vi "Session Daemon Async.vi"(9 "Engine Notifier":refnum<notifier>, 10 "TS License Type":T1, 11 "Dev Debug?":bool) -> ()   [LabVIEW 2020, in "TSnax.lvlib" / "Engine.lvclass"]
uses:
  Engine.lvclass
  TS License Type.ctl
  Daemon State.ctl
  UIMessage Callbacks.ctl
  UIMessage Callback.ctl
  UIMsg Callback VI.ctl
  UIMsg.ctl
  Ref Data.ctl
  PropertyObject/PropertyObject.lvclass
  SequenceFile/SequenceFile.lvclass
  Engine.lvclass/Engine.ctl
  SequenceFile Response.ctl
  VariableContainer Response.ctl
  Execution Response.ctl
  Execution/Execution.lvclass
  Report Response.ctl
  Report/Report.lvclass
  UIMessage/UIMessage.lvclass
  TSnax.lvlib
panel:
  out "Log":string
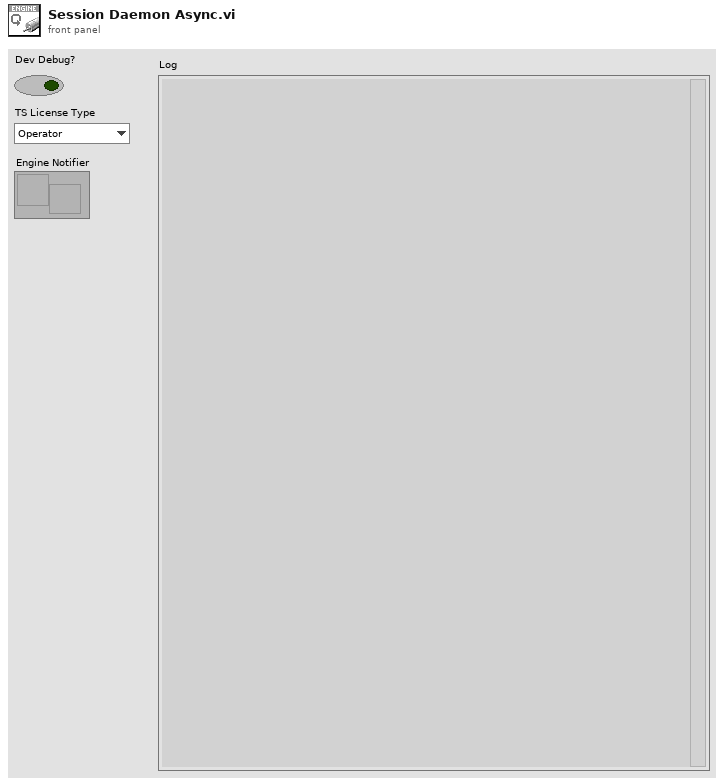
[diagram p1: front panel]
types:
  T1 = typedef "TSnax.lvlib/TS License Type.ctl" = enum16{"Operator", "CustomEditor", "SequenceEditor"}
  T2 = enum32{"invalid app kind", "Development System", "Run Time System", "Student Edition", "Embedded LabVIEW", "Evaluation", "Custom"}
  T3 = typedef "TSnax.lvlib/Engine.lvclass/Daemon State.ctl" = enum16{"Init", "Run", "Close"}
  T4 = typedef "TSnax.lvlib/Engine.lvclass/Ref Data.ctl" = cluster{"Station Globals":refnum<class "PropertyObject.lvclass">, "Station Model":refnum<class "SequenceFile.lvclass">, "Trace Delay":u32, "Execution Map":map{i32, refnum<class "Execution.lvclass">}}
  T5 = typedef "TSnax.lvlib/Engine.lvclass/UIMessage Callbacks.ctl" = cluster{"Callbacks":T6[], "ID Map":map{T8, i32[]}}
  T6 = typedef "TSnax.lvlib/Engine.lvclass/UIMessage Callback.ctl" = cluster{"VI":T7, "Owner":refnum<class>, "User Data":variant, "IDs":T8[]}
  T7 = typedef "TSnax.lvlib/Engine.lvclass/UIMsg Callback VI.ctl" = refnum<vi>
  T8 = typedef "TSnax.lvlib/UIMsg.ctl" = enum16{"Unknown", "BreakOnUserRequest", "BreakOnBreakpoint", "BreakOnRunTimeError", "Trace", "TerminatingExecution", "AbortingExecution", "KillingExecutionThreads", "EndExecution", "ShutDownComplete", "StartExecution", "ProgressPercent", "ProgressText", "StartInteractiveExecution", "EndInteractiveExecution", "TerminatingInteractiveExecution", "TerminationCancelled", "ResumeFromBreak", "StartFileExecution", "EndFileExecution", "ShutDownCancelled", "LocalizationSettingChanged", "OpenWindows", "TileWindows", "CascadeWindows", "ReportChanged", "CloseWindows", "RefreshWindows", "ClientFileChanged", "DisplayReport", "ModelState_Initializing", "ModelState_Waiting", "ModelState_Identified", "ModelState_BeginTesting", "ModelState_TestingComplete", "ModelState_PostProcessingComplete", "ModelState_EnabledStateSet", "ReportLocationChanged", "GotoLocation", "PushUndoItem", "OutputMessages", "TypePaletteFileListChanged", "NonTerminatingThreadsArePreventingTermination", "ModelState_PostProcessing", "ReportCollectionChanged", "RuntimeError"}
  T9 = enum32{"Invalid", "Standard", "Closed", "Hidden", "Minimized", "Maximized"}
  T10 = typedef "TSnax.lvlib/Engine.lvclass/SequenceFile Response.ctl" = cluster{"SequenceFile":refnum<class "SequenceFile.lvclass">, "Error":errorcluster}
  T11 = typedef "TSnax.lvlib/Engine.lvclass/VariableContainer Response.ctl" = cluster{"PropertyObject":refnum<class "PropertyObject.lvclass">, "Error":errorcluster}
  T12 = typedef "TSnax.lvlib/Engine.lvclass/Execution Response.ctl" = cluster{"Execution":refnum<class "Execution.lvclass">, "Error":errorcluster}
  T13 = typedef "TSnax.lvlib/Engine.lvclass/Report Response.ctl" = cluster{"Report":refnum<class "Report.lvclass">, "Error":errorcluster}
  T14 = typedef "TSnax.lvlib/File Load Options.ctl" = cluster{"Use Search Dirs? (T)":bool, "Conflict as Error? (T)":bool, "Check Station Model? (F)":bool, "Preload Modules? (T)":bool, "Skip Load Callback? (F)":bool, "Reload if Loaded? (F)":bool}
  T15 = typedef "TSnax.lvlib/Engine.lvclass/VariableContainer Type.ctl" = enum16{"StationGlobals", "TemporaryGlobals", "NewPropertyObject", "SubProperty"}
  T16 = typedef "TSnax.lvlib/Execution Options.ctl" = cluster{"Use Default Model (T)":bool, "Release Related References (T)":bool}
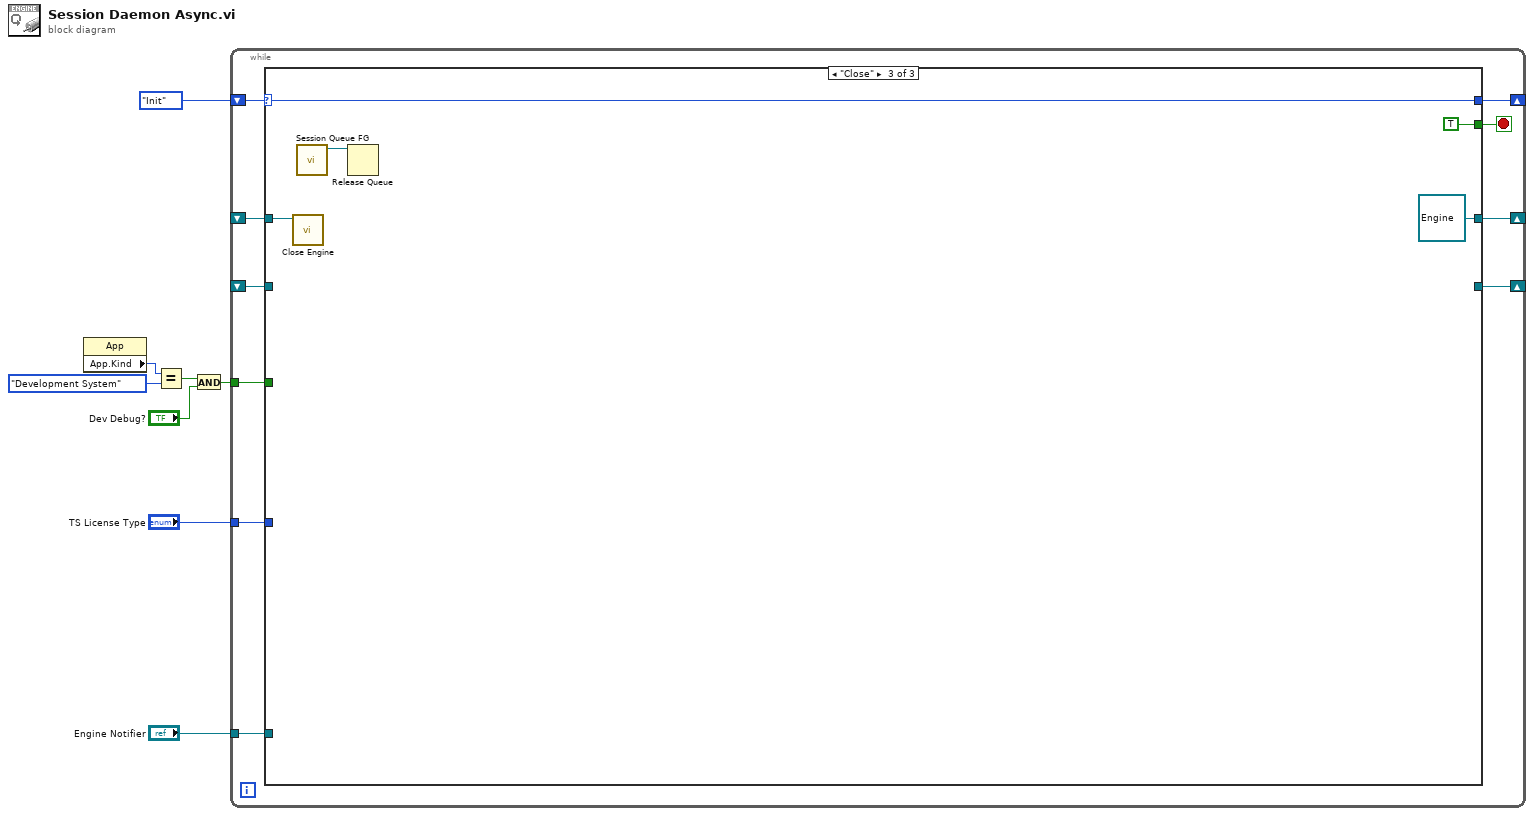
[diagram p0: block diagram]
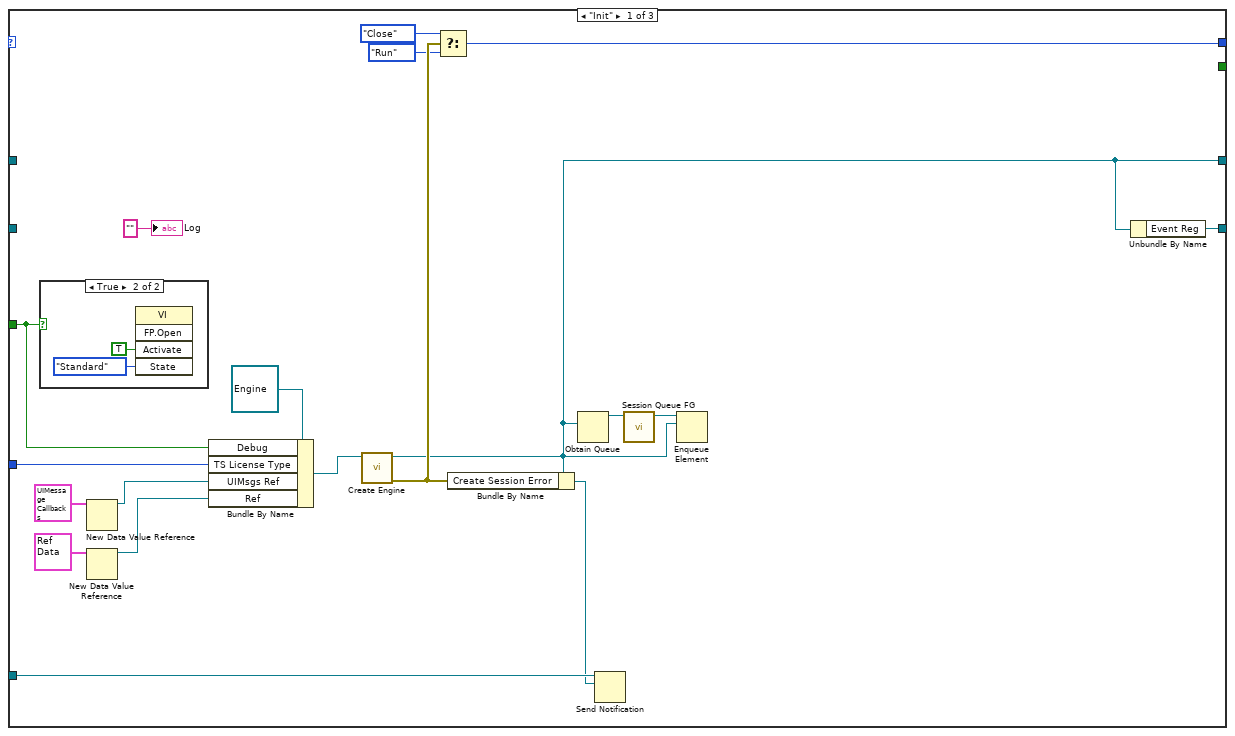
[diagram p2: hidden frame]
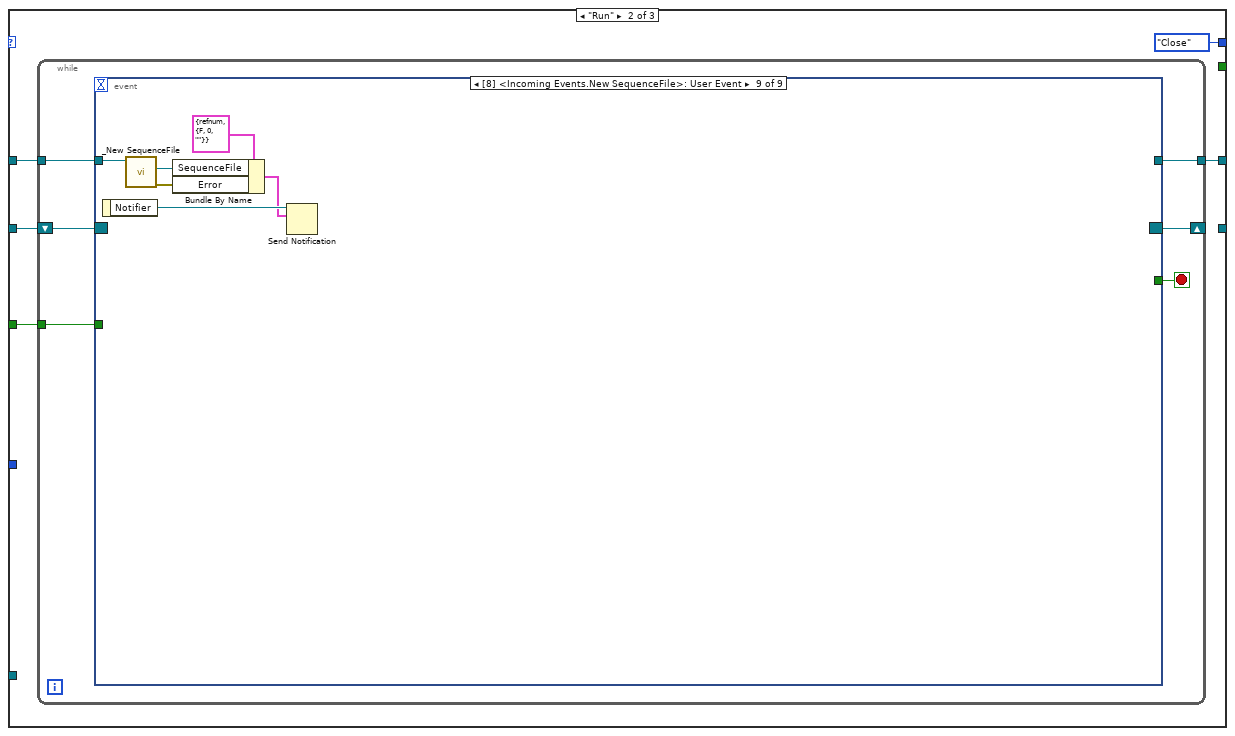
[diagram p4: hidden frame]
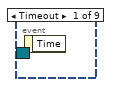
[diagram p5: hidden frame]
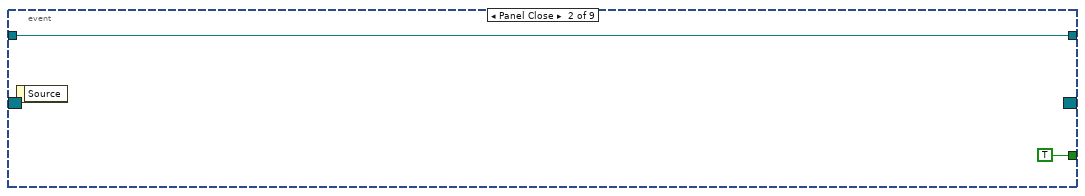
[diagram p6: hidden frame]
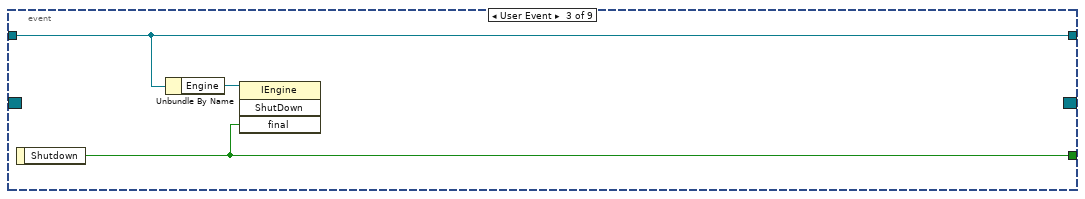
[diagram p7: hidden frame]
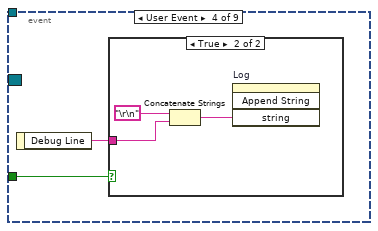
[diagram p8: hidden frame]
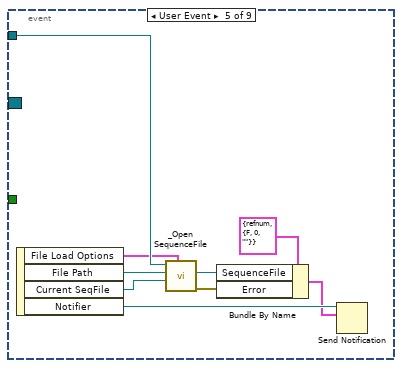
[diagram p10: hidden frame]
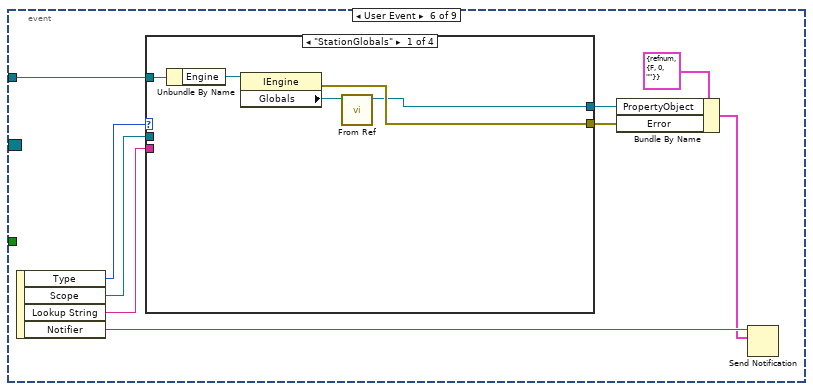
[diagram p11: hidden frame]
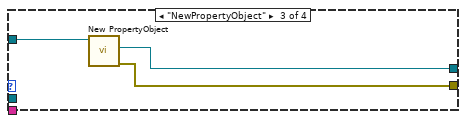
[diagram p13: hidden frame]
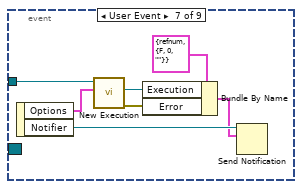
[diagram p15: hidden frame]
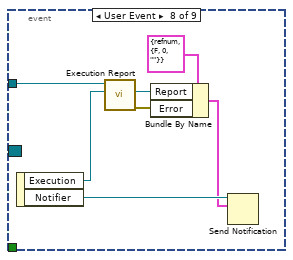
[diagram p16: hidden frame]
diagram:
  n1 = property class="App"() -> ("App.Kind"=w5:T2)  [unwired: 2 in, 2 out]
  n2 = Equal?(x=w5, y=T2."Development System") -> (x = y?=w3:bool)
  n3 = And(x=w3, y="Dev Debug?") -> (x .and. y?=w2:bool)
  n4 = while {
    shift-right: [w17] -> _
    shift-left: Daemon_State."Init" ("Daemon State") -> [w18]
    tunnel: "TS License Type" -> [w15]
    tunnel: "Engine Notifier" -> [w14]
    tunnel: w2 -> [w13]
    shift-right: [w12] -> _
    shift-left: _ -> [w11]
    shift-right: [w10] -> _
    shift-left: _ -> [w9]
    stop <- w16 stop-if-true
    n5 = case shown="\"Close\"" w18 {
      selector: w18 -> [_ _ w111]
      tunnel: [w30 Daemon_State."Close" ("Daemon State") w111] -> w17
      tunnel: [_ _ TRUE] -> w16
      tunnel: w15 -> [w35 _ _]
      tunnel: w14 -> [w33 _ _]
      tunnel: w13 -> [w28 w42 _]
      tunnel: [w24 w41 refnum<class "Engine.lvclass"> refnum ("Engine out")] -> w12
      tunnel: w11 -> [_ w43 w108]
      tunnel: [w27 _ _] -> w10
      tunnel: w9 -> [_ w40 _]
      frame "Init" {
        n6 = case shown="True" w28 {
          frame False {
          }
          frame True {
            n7 = invoke class="VI" method="FP.Open"("Activate"=TRUE ("Activate?"), "State"=T9."Standard") -> ()  [unwired: 3 in, 5 out]
          }
        }
        n8 = New Data Value Reference(data value=T5 {"Callbacks"=[], "ID Map"={}} ("UIMessage Callbacks")) -> (data value reference=w21:refnum<data-value>)  [unwired: 1 in, 1 out]
        n9 = New Data Value Reference(data value=T4 {"Station Globals"=refnum, "Station Model"=refnum, "Trace Delay"=0, "Execution Map"={}} ("Ref Data")) -> (data value reference=w19:refnum<data-value>)  [unwired: 1 in, 1 out]
        n10 = Bundle By Name(cluster=refnum<class "Engine.lvclass"> refnum ("TSnax.lvlib:Engine.lvclass"), "Debug"=w28, "TS License Type"=w35, "UIMsgs Ref"=w21, "Ref"=w19) -> (w34:refnum<class "Engine.lvclass">)
        n11 = call "Create Engine.vi"("Engine in"=w34) -> ("error out"=w37:errorcluster, "Engine out"=w24:refnum<class "Engine.lvclass">)  [unwired: 9 in]
        n12 = Select(t=Daemon_State."Close" ("Daemon State"), s=w37, f=Daemon_State."Run" ("Daemon State")) -> (s? t:f=w30:T3)
        n13 = Bundle By Name(cluster=w24, "Create Session Error"=w37) -> (w32:refnum<class "Engine.lvclass">)
        n14 = Obtain Queue(element data type=w24) -> (queue out=w26:refnum<queue>)  [unwired: 4 in, 2 out]
        n15 = Send Notification(notification=w32, notifier=w33) -> ()  [unwired: 1 in, 2 out]
        n16 = call "Session Queue FG.vi"("Session Queue In"=w26) -> ("Session Queue"=w25:refnum<queue>)  [unwired: 9 in, 1 out]
        n17 = Enqueue Element(queue=w25, element=w24) -> ()  [unwired: 2 in, 3 out]
        n18 = Unbundle By Name(w24) -> ("Event Reg"=w27:refnum<event-registration>)
        "Log" <- "" ("Log")
      }
      frame "Run" {
        n19 = while {
          tunnel: w43 -> [w50]
          tunnel: w42 -> [w49]
          tunnel: [w47] -> w41
          shift-right: [w45] -> _
          shift-left: w40 -> [w46]
          stop <- w48 stop-if-true
          n20 = event shown="[8] <Incoming Events.New SequenceFile>: User Event" {
            selector: w46 -> [_ _ _ _ _ _ _ _ _]
            dyn-events: [_ _ _ _ _ _ _ _ _] -> w45
            timeout: _ -> [_ _ _ _ _ _ _ _ _]
            tunnel: w50 -> [_ w51 w55 _ w69 w77 w93 w100 w106]
            tunnel: w49 -> [_ _ _ w56 _ _ _ _ _]
            tunnel: [_ TRUE w53 _ _ _ _ _ _] -> w48
            tunnel: [_ w51 w55 _ _ _ _ _ _] -> w47
            event Timeout {
              n21 = event-data() -> ()  [unwired: 1 in, 1 out]
            }
            event Panel Close {
              n22 = event-data() -> ()  [unwired: 1 in, 1 out]
            }
            event User Event {
              n23 = event-data() -> ("Shutdown"=w53:bool)  [unwired: 1 in]
              n24 = Unbundle By Name(w55) -> ("Engine"=w54:refnum<k7>)
              n25 = invoke class="IEngine" method="ShutDown"(reference=w54, "final"=w53) -> ()  [unwired: 2 in, 4 out]
            }
            event User Event {
              n26 = event-data() -> ("Debug Line"=w57:string)  [unwired: 1 in]
              n27 = case shown="True" w56 {
                tunnel: w57 -> [_ w59]
                frame False {
                }
                frame True {
                  n28 = Concatenate Strings("\r\n", w59) -> (w58:string)
                  n29 = invoke on="Log" class="Str" method="Append String"("string"=w58) -> ()  [unwired: 3 in, 4 out]
                }
              }
            }
            event User Event {
              n30 = event-data() -> ("File Load Options"=w67:T14, "File Path"=w68:path, "Current SeqFile"=w66:refnum<class "SequenceFile.lvclass">, "Notifier"=w65:refnum<notifier>)  [unwired: 1 in]
              n31 = call "_Open SequenceFile.vi"("File Load Options"=w67, "Current SeqFile"=w66, "File Path"=w68, "Engine in"=w69) -> ("error out"=w61:errorcluster, "SequenceFile"=w62:refnum<class "SequenceFile.lvclass">)  [unwired: 6 in]
              n32 = Bundle By Name(cluster=T10 {"SequenceFile"=refnum, "Error"={"status"=FALSE, "code"=0, "source"=""}} ("notification"), "SequenceFile"=w62, "Error"=w61) -> (w63:T10)
              n33 = Send Notification(notification=w63, notifier=w65) -> ()  [unwired: 1 in, 2 out]
            }
            event User Event {
              n34 = event-data() -> ("Type"=w78:T15, "Scope"=w76:refnum<class "PropertyObject.lvclass">, "Lookup String"=w75:string, "Notifier"=w74:refnum<notifier>)  [unwired: 1 in]
              n35 = case shown="\"StationGlobals\"" w78 {
                tunnel: w77 -> [w83 _ w86 _]
                tunnel: w76 -> [_ _ _ _]
                tunnel: w75 -> [_ _ _ _]
                tunnel: [w79 _ w85 _] -> w71
                tunnel: [w80 _ w84 _] -> w70
                frame "StationGlobals" {
                  n36 = Unbundle By Name(w83) -> ("Engine"=w82:refnum<k7>)
                  n37 = property class="IEngine"(reference=w82) -> (error out=w80:errorcluster, "Globals"=w81:refnum<k7>)  [unwired: 1 in, 1 out]
                  n38 = call "From Ref.vi"("PropertyObject"=w81) -> ("PropertyObject out"=w79:refnum<class "PropertyObject.lvclass">)  [unwired: 9 in, 1 out]
                }
                frame "TemporaryGlobals" {
                }
                frame "NewPropertyObject" {
                  n39 = call "New PropertyObject.vi"("Engine in"=w86) -> ("error out"=w84:errorcluster, "PropertyObject"=w85:refnum<class "PropertyObject.lvclass">)  [unwired: 8 in, 1 out]
                }
                frame "SubProperty" {
                }
              }
              n40 = Bundle By Name(cluster=T11 {"PropertyObject"=refnum, "Error"={"status"=FALSE, "code"=0, "source"=""}} ("notification"), "PropertyObject"=w71, "Error"=w70) -> (w72:T11)
              n41 = Send Notification(notification=w72, notifier=w74) -> ()  [unwired: 1 in, 2 out]
            }
            event User Event {
              n42 = event-data() -> ("Options"=w92:T16, "Notifier"=w88:refnum<notifier>)  [unwired: 1 in]
              n43 = call "New Execution.vi"("Execution Options"=w92, "Engine in"=w93) -> ("error out"=w89:errorcluster, "Execution"=w90:refnum<class "Execution.lvclass">)  [unwired: 7 in, 1 out]
              n44 = Bundle By Name(cluster=T12 {"Execution"=refnum, "Error"={"status"=FALSE, "code"=0, "source"=""}} ("Execution Response"), "Execution"=w90, "Error"=w89) -> (w87:T12)
              n45 = Send Notification(notification=w87, notifier=w88) -> ()  [unwired: 1 in, 2 out]
            }
            event User Event {
              n46 = event-data() -> ("Execution"=w99:refnum<class "Execution.lvclass">, "Notifier"=w98:refnum<notifier>)  [unwired: 1 in]
              n47 = call "Execution Report.vi"("Execution"=w99, "Engine in"=w100) -> ("error out"=w94:errorcluster, "Report"=w95:refnum<class "Report.lvclass">)  [unwired: 7 in, 1 out]
              n48 = Bundle By Name(cluster=T13 {"Report"=refnum, "Error"={"status"=FALSE, "code"=0, "source"=""}} ("notification"), "Report"=w95, "Error"=w94) -> (w96:T13)
              n49 = Send Notification(notification=w96, notifier=w98) -> ()  [unwired: 1 in, 2 out]
            }
            event User Event {
              n50 = event-data() -> ("Notifier"=w105:refnum<notifier>)  [unwired: 1 in]
              n51 = call "_New SequenceFile.vi"("Engine in"=w106) -> ("error out"=w102:errorcluster, "New SequenceFile"=w101:refnum<class "SequenceFile.lvclass">)  [unwired: 8 in, 1 out]
              n52 = Bundle By Name(cluster=T10 {"SequenceFile"=refnum, "Error"={"status"=FALSE, "code"=0, "source"=""}} ("notification"), "SequenceFile"=w101, "Error"=w102) -> (w103:T10)
              n53 = Send Notification(notification=w103, notifier=w105) -> ()  [unwired: 1 in, 2 out]
            }
          }
        }
      }
      frame "Close" {
        n54 = call "Close Engine.vi"("Engine in"=w108) -> ()  [unwired: 10 in, 1 out]
        n55 = call "Session Queue FG.vi"() -> ("Session Queue"=w107:refnum<queue>)  [unwired: 10 in, 1 out]
        n56 = Release Queue(queue=w107) -> ()  [unwired: 2 in, 3 out]
      }
    }
  }
